vi "IO Channel Name Collision Check.vi"() -> (0 "Channel Names Collide":bool)   [LabVIEW 2013]
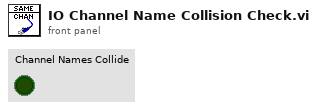
[diagram p1: front panel]
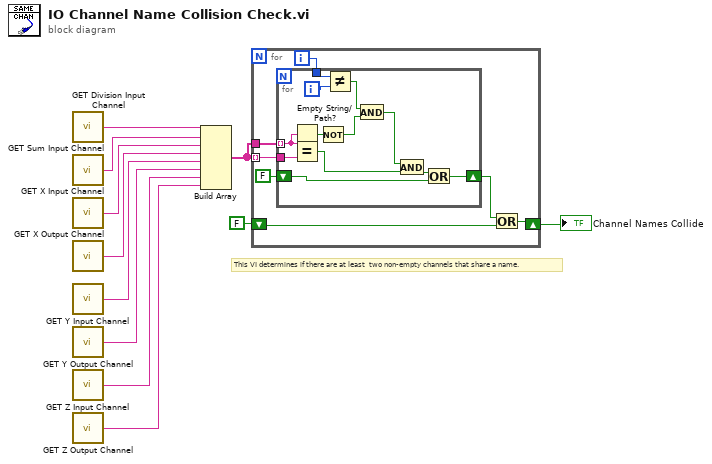
[diagram p0: block diagram]
diagram:
  # "This VI determines if there are at least  two non-empty channels that share a name."
  n1 = call "GET Division Input Channel.vi"() -> ("Division Input Channel"=w11:string)
  n2 = call "GET Sum Input Channel.vi"() -> ("Sum Input Channel"=w10:string)
  n3 = call "GET X Input Channel.vi"() -> ("X Input Channel"=w9:string)
  n4 = call "GET X Output Channel.vi"() -> ("X Output Channel"=w8:string)
  n5 = call "GET Y Input Channel.vi"() -> ("Y Input Channel"=w7:string)
  n6 = call "GET Y Output Channel.vi"() -> ("Y Output Channel"=w6:string)
  n7 = call "GET Z Input Channel.vi"() -> ("Z Input Channel"=w5:string)
  n8 = call "GET Z Output Channel.vi"() -> ("Z Output Channel"=w4:string)
  n9 = Build Array(w11, w10, w9, w8, w7, w6, w5, w4) -> (w3:string[])
  n10 = for {
    tunnel: w3 -> [w17] mode=indexing
    tunnel: w3 -> [w18]
    shift-right: [w14] -> w1
    shift-left: FALSE -> [w13]
    i -> [w12]
    n11 = for {
      tunnel: w18 -> [w23] mode=indexing
      tunnel: w17 -> [w30]
      shift-right: [w29] -> w15
      shift-left: FALSE -> [w28]
      tunnel: w12 -> [w27]
      i -> [w26]
      n12 = Empty String/Path?(string/path=w23) -> (empty?=w22:bool)
      n13 = Equal?(x=w23, y=w30) -> (x = y?=w24:bool)
      n14 = Not(x=w22) -> (.not. x?=w21:bool)
      n15 = Not Equal?(x=w27, y=w26) -> (x != y?=w20:bool)
      n16 = And(x=w20, y=w21) -> (x .and. y?=w19:bool)
      n17 = And(x=w19, y=w24) -> (x .and. y?=w25:bool)
      n18 = Or(x=w25, y=w28) -> (x .or. y?=w29:bool)
    }
    n19 = Or(x=w15, y=w13) -> (x .or. y?=w14:bool)
  }
  "Channel Names Collide" <- w1
